vi "DequeueWithParameters.vi"(8 "error in":errorcluster, 11 "Queue in":refnum<queue>) -> (0 "error out":errorcluster, 1 "channelStr":string, 2 "command":string, 3 "Queue out":refnum<queue>, 4 "telegram":string, 5 "channel":i32, 7 "QueueCmd":string)   [LabVIEW 2018]
doc: "Syntax for enqueue: command;[channel];[telegram]"
panel:
  # "Dequeue with Parameters"
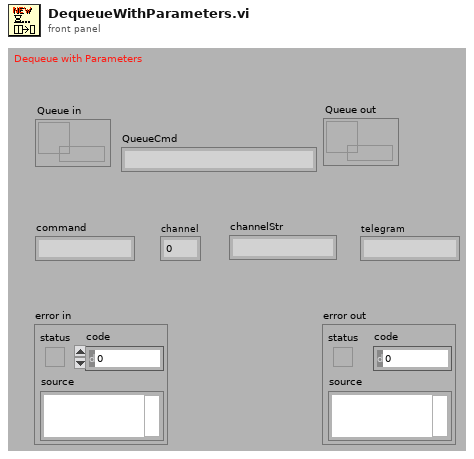
[diagram p1: front panel]
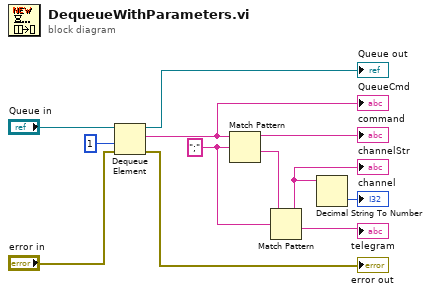
[diagram p0: block diagram]
diagram:
  w7 = ";" ("dev_char")
  n1 = Dequeue Element(queue="Queue in", timeout in ms (-1)=1, error in (no error)="error in") -> (queue out=→"Queue out":refnum<queue>, element=w1:string, error out=→"error out":errorcluster)  [unwired: 1 out]
  "QueueCmd" <- w1
  n2 = Match Pattern(string=w1, regular expression=w7) -> (before substring=→"command":string, after substring=w5:string)  [unwired: 3 out]
  n3 = Match Pattern(string=w5, regular expression=w7) -> (before substring=w2:string, after substring=→"telegram":string)  [unwired: 3 out]
  "channelStr" <- w2
  n4 = Decimal String To Number(string=w2) -> (number=→"channel":i32)  [unwired: 3 out]
